vi "Test Time Measurement.vi"() -> (0 "VI Tester Testing time (seconds)":dbl, 1 "Caraya Testing time (seconds)":dbl, 2 "ICov Testing time (seconds)":dbl, 3 "UTF Testing time (seconds)":dbl)   [LabVIEW 2018]
uses:
  <vilib>/utf/common/utf_test_result.ctl
  Caraya Time Measurement.vi
  <vilib>/utf/NI_UnitTestFramework.lvlib
panel:
  out "Caraya report":string
  out "Caraya In Progress":bool
  out "VI Tester report":string
  out "VI Tester In Progress":bool
  out "ICov Results":enum16{"PASSED", "FAILED", "ERROR"}[](array[ring])
  out "ICov In Progress":bool
  out "UTF In Progress":bool
  out "UTF Results":T1[](array[typedef])
  # "UTF"
  # "VI Tester"
  # "ICov"
  # "Caraya"
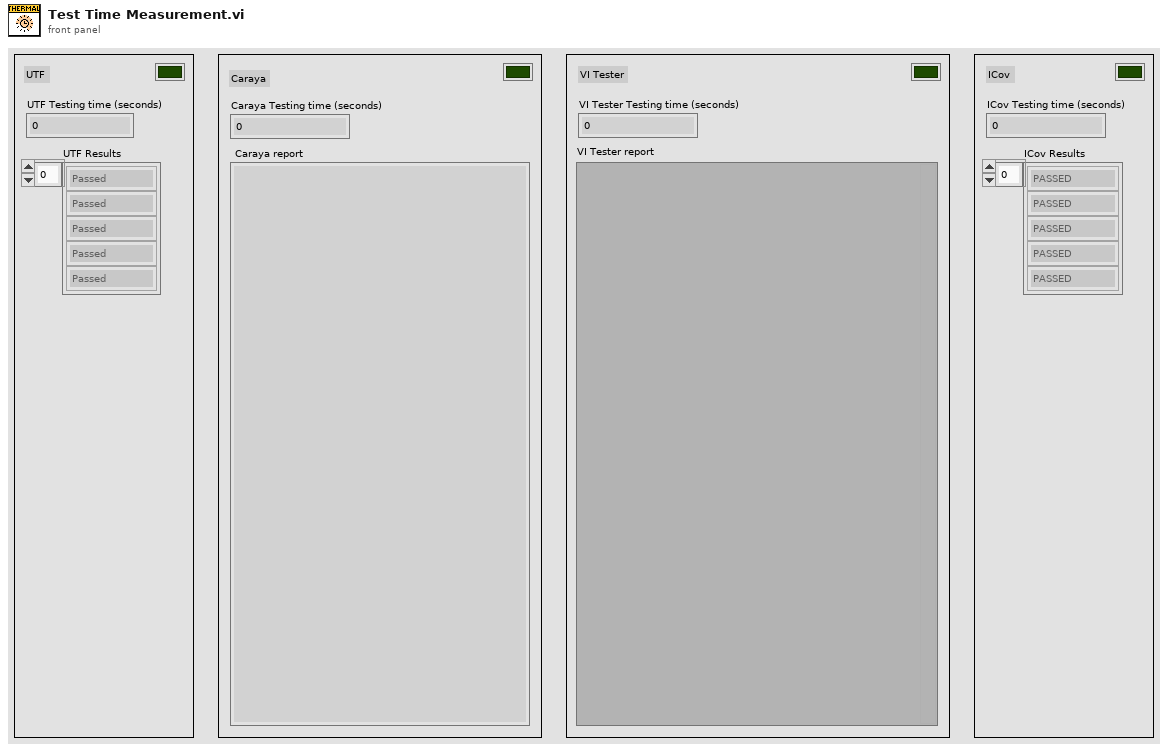
[diagram p1: front panel]
types:
  T1 = typedef "NI_UnitTestFramework.lvlib/utf_test_result.ctl" = enum16{"Passed", "Failed", "Error", "Skipped", "Not Processed"}
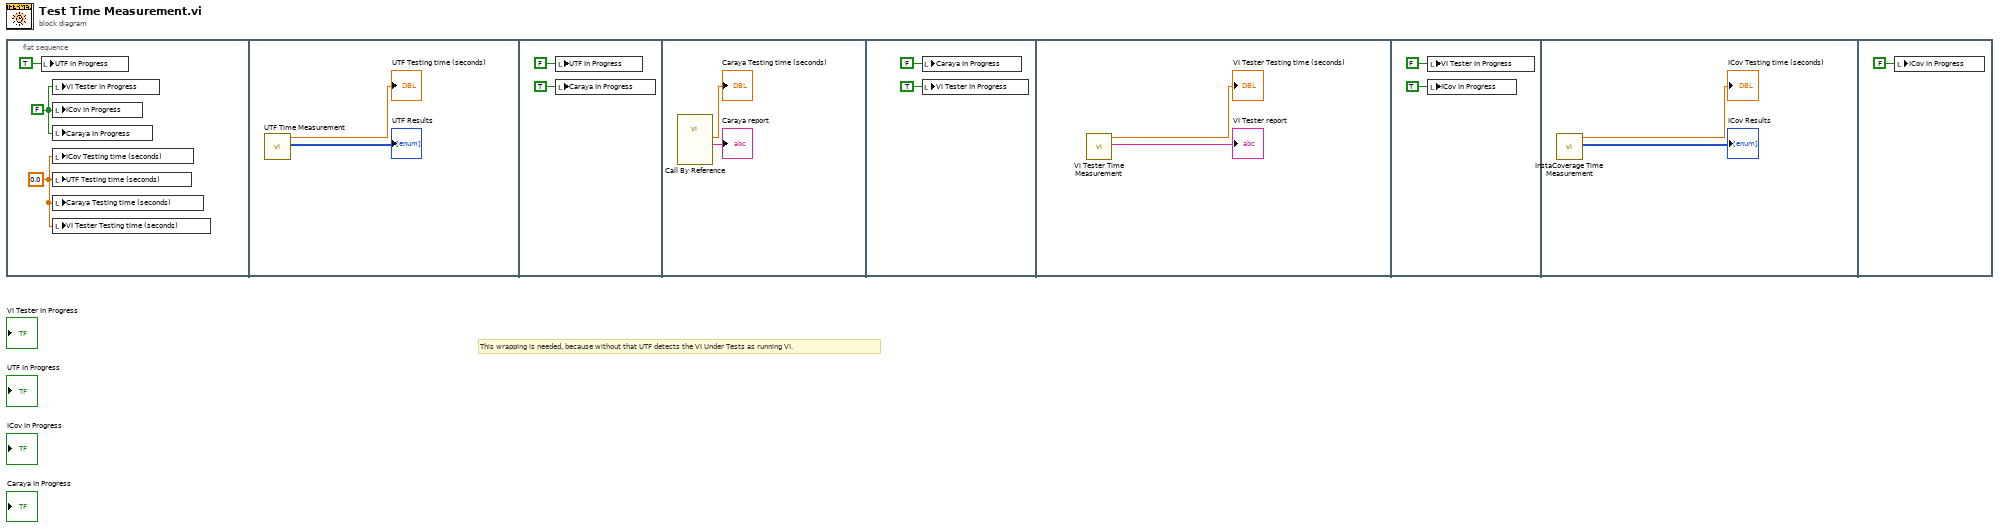
[diagram p0: block diagram]
diagram:
  # "This wrapping is needed, because without that UTF detects the VI Under Tests as running VI."
  n1 = flat-sequence {
    frame #0 {
      w2 = FALSE
      w1 = 0.0
      n2 = local write "UTF In Progress"(TRUE) -> ()
      n3 = local write "VI Tester In Progress"(w2) -> ()
      n4 = local write "ICov In Progress"(w2) -> ()
      n5 = local write "Caraya In Progress"(w2) -> ()
      n6 = local write "ICov Testing time (seconds)"(w1) -> ()
      n7 = local write "UTF Testing time (seconds)"(w1) -> ()
      n8 = local write "Caraya Testing time (seconds)"(w1) -> ()
      n9 = local write "VI Tester Testing time (seconds)"(w1) -> ()
    }
    frame #1 {
      n10 = call "UTF Time Measurement.vi"() -> ("UTF Results"=→"UTF Results":T1[], "UTF Testing time (seconds)"=→"UTF Testing time (seconds)":dbl)  [unwired: 10 in]
    }
    frame #2 {
      n11 = local write "UTF In Progress"(FALSE) -> ()
      n12 = local write "Caraya In Progress"(TRUE) -> ()
    }
    frame #3 {
      n13 = call-by-ref "?"() -> ("Caraya report"=→"Caraya report":string, "ICov Testing time (seconds)"=→"Caraya Testing time (seconds)":dbl)  [unwired: 12 in, 2 out]
    }
    frame #4 {
      n14 = local write "Caraya In Progress"(FALSE) -> ()
      n15 = local write "VI Tester In Progress"(TRUE) -> ()
    }
    frame #5 {
      n16 = call "Vi Tester Time Measurement.vi"() -> ("VI Tester report"=→"VI Tester report":string, "VI Tester Testing time (seconds)"=→"VI Tester Testing time (seconds)":dbl)  [unwired: 10 in]
    }
    frame #6 {
      n17 = local write "VI Tester In Progress"(FALSE ("ICov In Progress")) -> ()
      n18 = local write "ICov In Progress"(TRUE ("ICov In Progress")) -> ()
    }
    frame #7 {
      n19 = call "InstaCoverage Time Measurement.vi"() -> ("ICov Results"=→"ICov Results":enum16{"PASSED", "FAILED", "ERROR"}[], "ICov Testing time (seconds)"=→"ICov Testing time (seconds)":dbl)  [unwired: 10 in]
    }
    frame #8 {
      n20 = local write "ICov In Progress"(FALSE ("ICov In Progress")) -> ()
    }
  }
